vi "tearDown.vi"(8 "error in (no error)":errorcluster, 11 "reference in":refnum<class "SMO.UI_TestCase.lvclass">) -> (0 "error out":errorcluster, 3 "reference out":refnum<class "SMO.UI_TestCase.lvclass">)   [LabVIEW 2013, in "SMO.UI_TestCase.lvclass"]
doc: "tearDown runs after the test method has completed. Use this method to clean up any operations or references that were opened by setUp or the test method. Unit tests should be independent of other unit tests so this VI should ensure that the next test can run in a 'clean' test environment."
uses:
  SMO.UI_TestCase.lvclass
  SMO.UI_TestCase.lvclass/SMO.UI_TestCase.ctl
  Projects/JKI SMO Git/JKI-State-Machine-Objects/src/SMO/SMO.lvclass
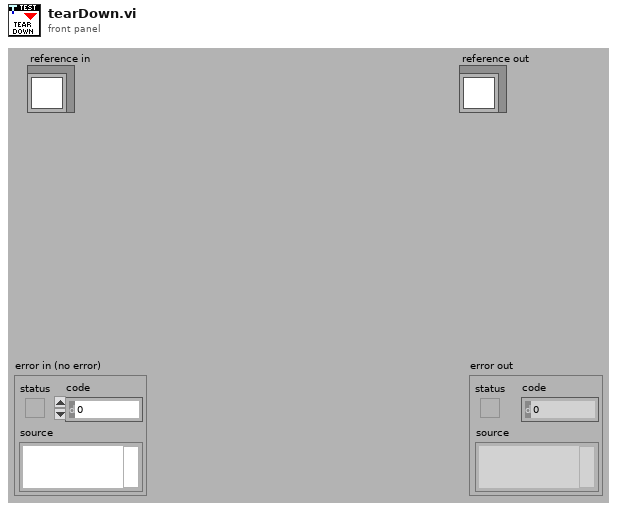
[diagram p1: front panel]
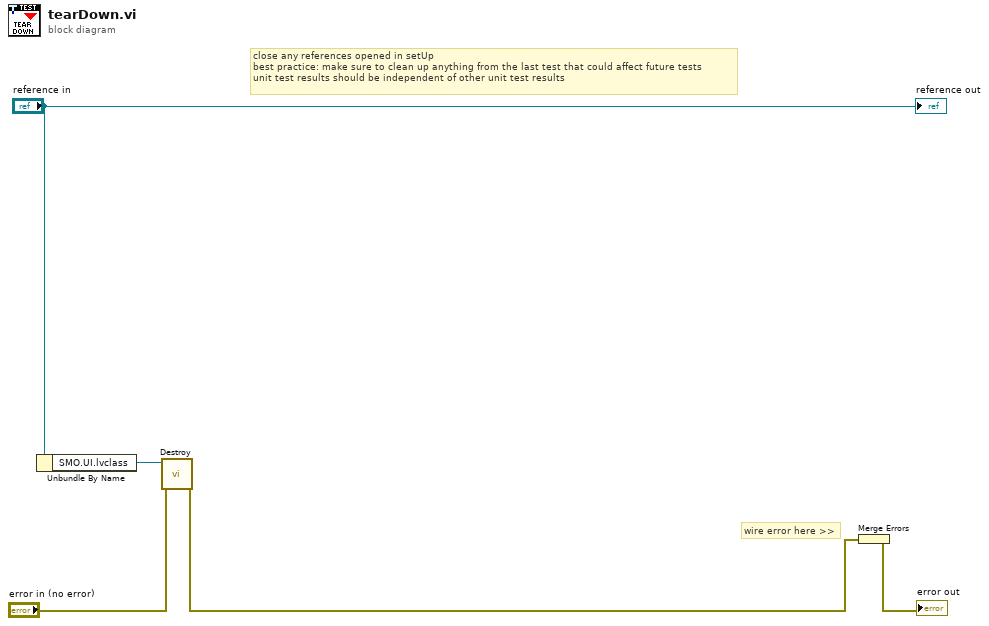
[diagram p0: block diagram]
diagram:
  # "wire error here >>"
  # "close any references opened in setUp\nbest practice: make sure to clean up anything from the last test that could affect future tests\nunit test results should be independent of other unit test results"
  n1 = Unbundle By Name("reference in") -> ("SMO.UI.lvclass"=w3:refnum<class "SMO.UI.lvclass">)
  n2 = call "Destroy.vi"("error in (no error)"="error in (no error)", "SMO"=w3) -> ("error out"=w1:errorcluster)  [unwired: 9 in]
  n3 = Merge Errors(w1) -> (→"error out":errorcluster)
  "reference out" <- "reference in"
